vi "Put.vi"() -> ()   [LabVIEW 2020]
uses:
  <vilib>/httpClient/PUTBuffer.vi
  <vilib>/httpClient/LabVIEWHTTPClient.lvlib
panel:
  in  "Data":cluster{"name":string, "job":string}={"name"="Jane Doe", "job"="Project Manager"}
  out "error out":errorcluster
  out "body":string
  out "headers":string
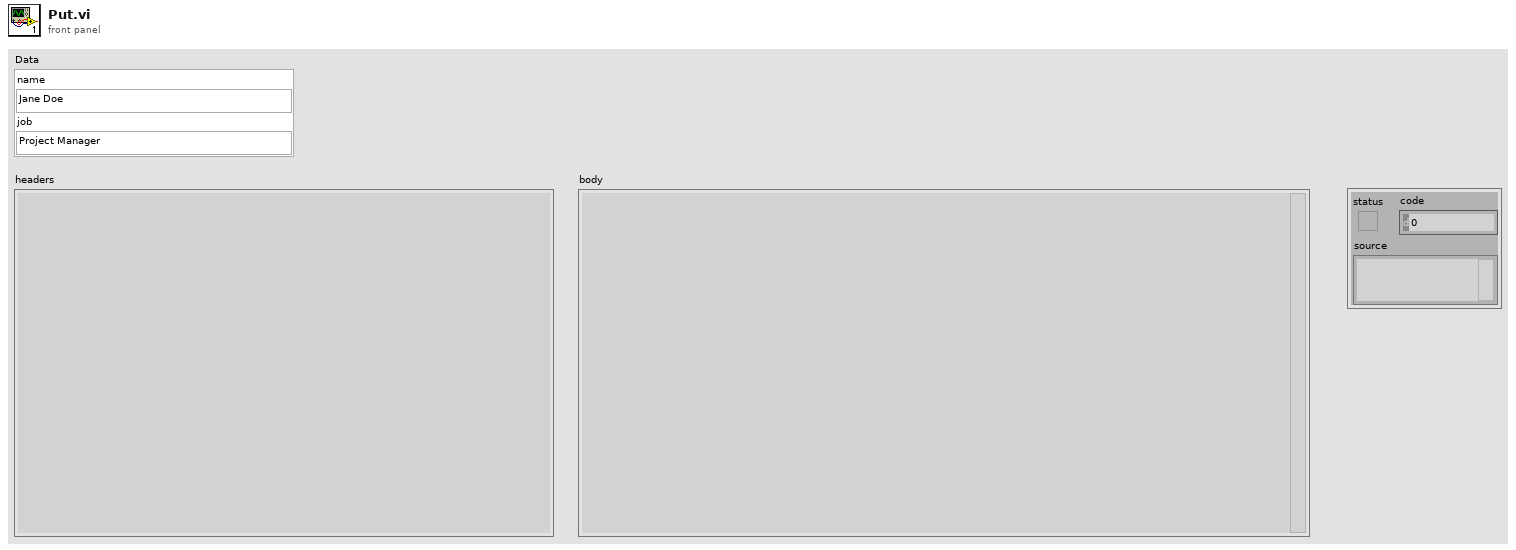
[diagram p1: front panel]
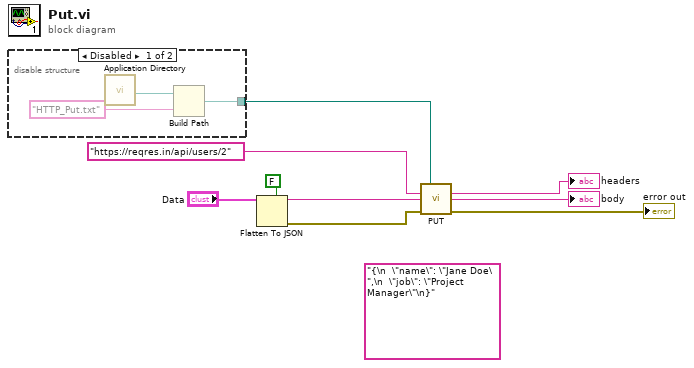
[diagram p0: block diagram]
diagram:
  (unwired) "{\n  \"name\": \"Jane Doe\",\n  \"job\": \"Project Manager\"\n}" ("buffer")
  n1 = disable-structure shown="Disabled" {
    disable-tunnel: [w10 _] -> w8
    frame Disabled {
      n2 = call <vilib>:"Application Directory.vi"() -> ("Application Directory"=w12:path)
      n3 = Build Path(base path=w12, name or relative path="HTTP_Put.txt") -> (appended path=w10:path)
    }
    frame Enabled {
    }
  }
  n4 = Flatten To JSON(enable LabVIEW extensions? (T)=FALSE, anything="Data") -> (JSON string=w5:string, 11:w3:errorcluster)  [unwired: 1 in]
  n5 = call-poly <vilib>:"PUT.vi"("output file"=w8, "url"="https://reqres.in/api/users/2", "buffer"=w5, "error in (no error)"=w3) -> ("headers"=→"headers":string, "body"=→"body":string, "error out"=→"error out":errorcluster)  [unwired: 8 in, 1 out]
